vi "FeedbackDecode_CheckPupilConnection.vi"() -> (0 "Connected?":bool)   [LabVIEW 2020]
uses:
  <vilib>/regexp/Match Regular Expression.xnode
panel:
  out "standard output":string
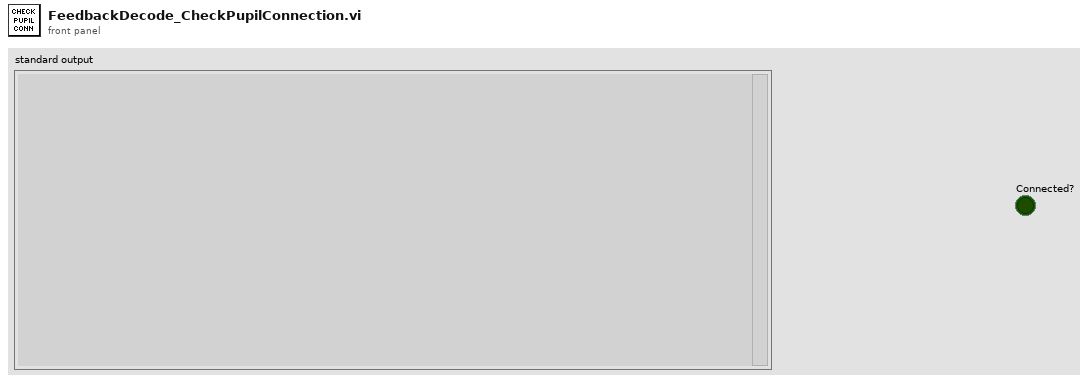
[diagram p1: front panel]
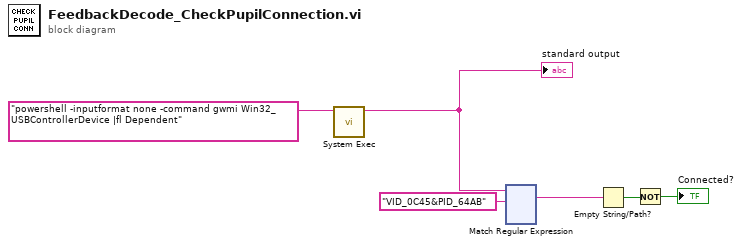
[diagram p0: block diagram]
diagram:
  n1 = call <vilib>:"System Exec.vi"("command line"="powershell -inputformat none -command gwmi Win32_USBControllerDevice |fl Dependent") -> ("standard output"=w5:string)  [unwired: 7 in, 3 out]
  "standard output" <- w5
  n2 = xnode "Match Regular Expression"("input string"=w5, "regular expression"="VID_0C45&PID_64AB") -> ("whole match"=w3:string)  [unwired: 4 in, 4 out]
  n3 = Empty String/Path?(string/path=w3) -> (empty?=w2:bool)
  n4 = Not(x=w2) -> (.not. x?=→"Connected?":bool)
